vi "GetComments.vi"(8 "error in":errorcluster, 11 "Defect in":refnum<class "Defect.lvclass">) -> (0 "error out":errorcluster, 2 "Comments":refnum<class "UserComment.lvclass">[](array[class]), 3 "Defect out":refnum<class "Defect.lvclass">)   [LabVIEW 2021, in "ProligentXMLGenerator.lvlib" / "Defect.lvclass"]
doc: "Represents comments made by a user. Note that a user comment is considered unique when the comment, user and time are equal for a given associated fact. For example, if two failures have the same comment, user and time, they will be considered as two different comments because they are not attached to the same failure. But if two xmls are received by the DIT and they contain the same comment, user and time for the same failure ID, then they will be considered the same comment and the second comment will be discarded silently by the DIT."
uses:
  Defect.lvclass
  Defect.lvclass/Defect.ctl
  Model/UserComment/UserComment.lvclass
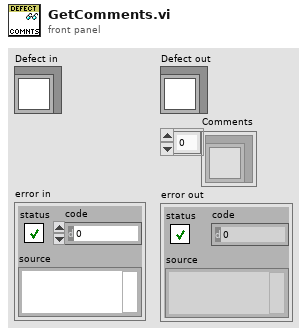
[diagram p1: front panel]
types:
  T1 = typedef "ProligentXMLGenerator.lvlib/Defect.lvclass/Data.ctl" = cluster{"Name":string, "Comments":refnum<class "UserComment.lvclass">[], "CustomData":refnum<class "CustomData.lvclass">, "DefectId":refnum<class "Guid.lvclass">, "OpenTime":refnum<class "DateTime.lvclass">, "TimeZoneInfoId":string}
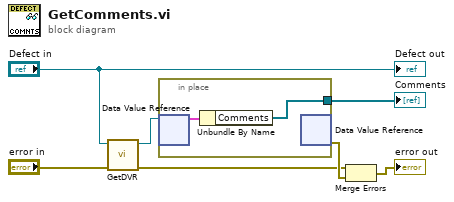
[diagram p0: block diagram]
diagram:
  n1 = call "GetDVR.vi"("error in"="error in", "Defect"="Defect in") -> ("error out"=w1:errorcluster, "DVRReference"=w6:refnum<data-value>)  [unwired: 8 in]
  n2 = in-place "In Place Element Structure" {
    in-place-border: [w8] -> w2
    n3 = in-place-dvr #1(w6) -> (w9:T1)  [unwired: 1 out]
    n4 = Unbundle By Name(w9) -> ("Comments"=w8:refnum<class "UserComment.lvclass">[])
    n5 = in-place-dvr #1() -> (w7:errorcluster)  [unwired: 1 in, 1 out]
  }
  "Comments" <- w2
  n6 = Merge Errors(w1, w7) -> (→"error out":errorcluster)
  "Defect out" <- "Defect in"
